vi "gps simul.vi"() -> ()   [LabVIEW 2016]
panel:
  in  "borrar trayectoria":bool
  in  "detener":bool
  in  "capturar":bool
  out "trayectoria":cluster{dbl[], dbl[]}(graph)
  out "posicion":cluster{dbl[], dbl[]}(graph)
  in  "longitud":dbl(slide) scale=-180.0..180.0
  in  "latitud":dbl(slide) scale=-90.0..90.0
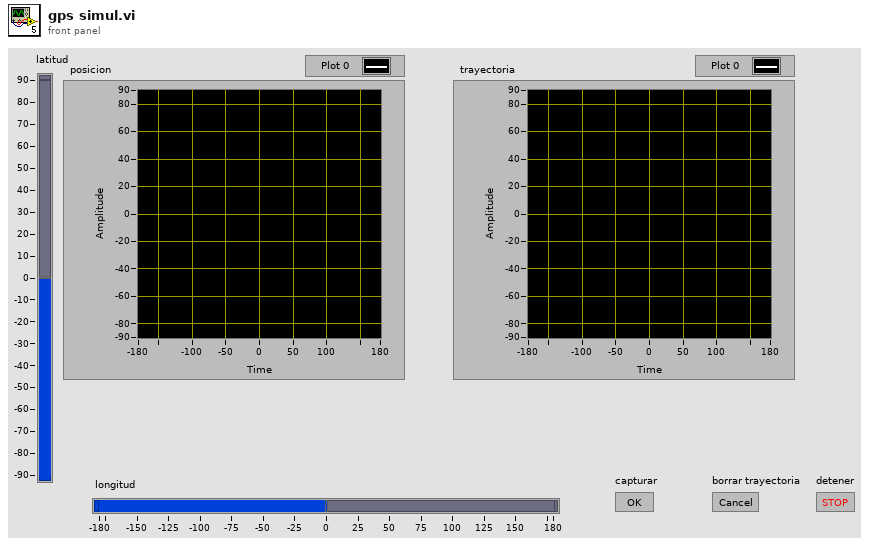
[diagram p1: front panel]
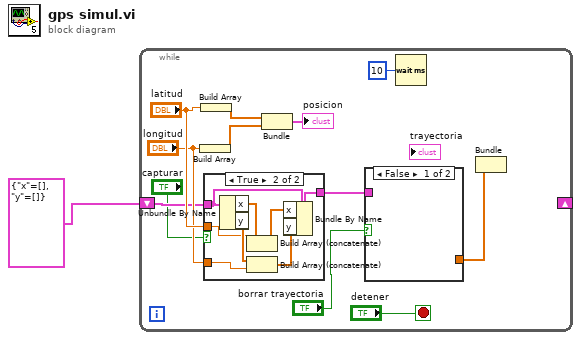
[diagram p0: block diagram]
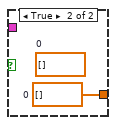
[diagram p2: hidden frame]
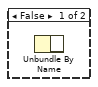
[diagram p3: hidden frame]
diagram:
  n1 = while {
    shift-right: _ -> [_]
    shift-left: cluster{"x":dbl[], "y":dbl[]} {"x"=[], "y"=[]} -> [w6]
    stop <- "detener" stop-if-true
    n2 = Build Array("longitud") -> (w10:dbl[])
    n3 = Build Array("latitud") -> (w9:dbl[])
    n4 = case shown="True" "capturar" {
      tunnel: "latitud" -> [_ w19]
      tunnel: "longitud" -> [_ w22]
      tunnel: w6 -> [_ w18]
      tunnel: [_ w17] -> w2
      frame False {
        n5 = Unbundle By Name() -> ()  [unwired: 1 in, 1 out]
      }
      frame True {
        n6 = Unbundle By Name(w18) -> ("x"=w21:dbl[], "y"=w20:dbl[])
        n7 = Build Array (concatenate)(w21, w19) -> (w16:dbl[])
        n8 = Build Array (concatenate)(w20, w22) -> (w15:dbl[])
        n9 = Bundle By Name(cluster=w18, "x"=w16, "y"=w15) -> (w17:cluster{"x":dbl[], "y":dbl[]})
      }
    }
    n10 = Bundle(w9, w10) -> (→"posicion":cluster{dbl[], dbl[]})  [unwired: 1 in]
    n11 = case shown="False" "borrar trayectoria" {
      tunnel: [_ w14] -> w3
      tunnel: w2 -> [_ _]
      frame False {
      }
      frame True {
        w14 = dbl[] []  # 0
        (unwired) dbl[] []  # 0
      }
    }
    n12 = Wait (ms)(milliseconds to wait=u32 10) -> ()  [unwired: 1 out]
    n13 = Bundle("0"=w3) -> ()  [unwired: 2 in, 1 out]
  }
